vi "Configure Number of Points.vi"(8 "error in (no error)":errorcluster, 10 "Number of Point":i32, 11 "VNA-Ag87xx in":refnum<class "VNA-Ag87xx.lvclass">) -> (0 "error out":errorcluster, 3 "VNA-Ag87xx out":refnum<class "VNA-Ag87xx.lvclass">)   [LabVIEW 2020, in "VNA-Ag87xx.lvclass"]
doc: "Configures the number of points in the sweep.\nThe number of points will be choosen to the nearest supported."
uses:
  VNA-Ag87xx.lvclass
  C:/Sandbox/Git_Sandbox/WiSpry Test Framework source code (LV20)/WiSpry Test Framework/Instruments/Instrument.lvclass
  C:/Sandbox/Git_Sandbox/WiSpry Test Framework source code (LV20)/WiSpry Test Framework/Instruments/Vector Network Analyzer/Vector Network Analyzer.lvclass
  Instrument.lvclass/Instrument.ctl
  Vector Network Analyzer.lvclass/Vector Network Analyzer.ctl
  Instrument.lvclass
  Vector Network Analyzer.lvclass
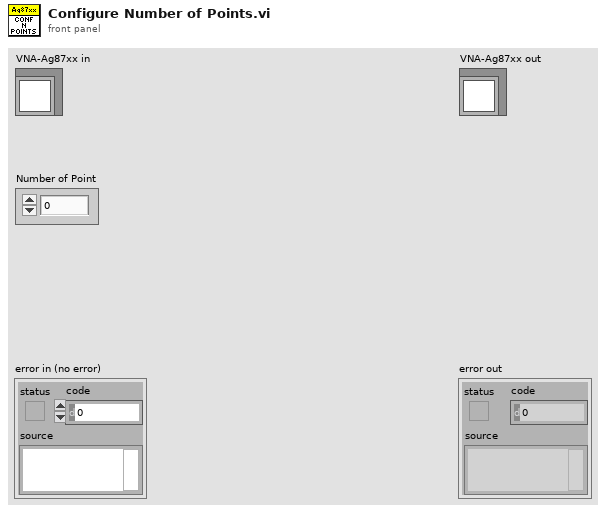
[diagram p1: front panel]
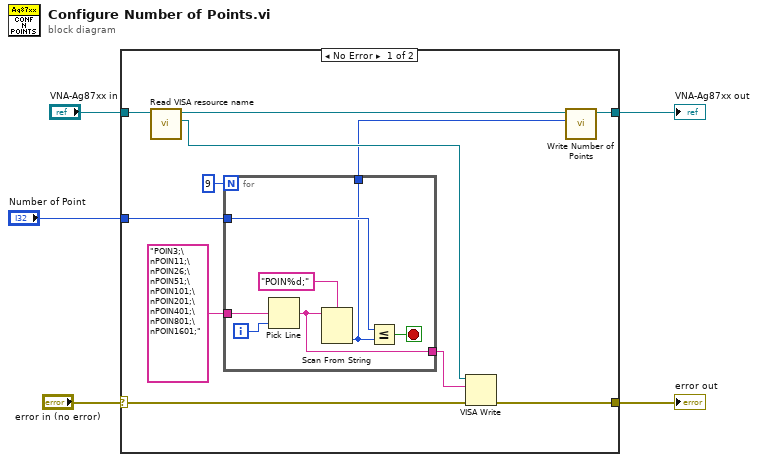
[diagram p0: block diagram]
diagram:
  n1 = case shown="No Error" "error in (no error)" {
    selector: "error in (no error)" -> [w13 w24]
    tunnel: [w10 w25] -> w3
    tunnel: "VNA-Ag87xx in" -> [w16 w25]
    tunnel: [w14 w24] -> w2
    tunnel: "Number of Point" -> [w9 _]
    frame No Error {
      n2 = call "Read VISA resource name.vi"("Instrument in"=w16) -> ("VISA resource name"=w12:refnum<visa-resource-name>, "Instrument out"=w11:refnum<class "VNA-Ag87xx.lvclass">)  [unwired: 9 in]
      n3 = for {
        N: 9 -> [_]
        tunnel: "POIN3;\nPOIN11;\nPOIN26;\nPOIN51;\nPOIN101;\nPOIN201;\nPOIN401;\nPOIN801;\nPOIN1601;" -> [w23]
        tunnel: w9 -> [w20]
        tunnel: [w17] -> w6
        tunnel: [w18] -> w7
        i -> [w22]
        stop <- w19 stop-if-true
        n4 = Pick Line(multi-line string=w23, line index=w22) -> (output string=w17:string)  [unwired: 1 in]
        n5 = Scan From String(format string="POIN%d;", input string=w17) -> (output 1=w18:i32)  [unwired: 3 in, 3 out]
        n6 = Less Or Equal?(x=w20, y=w18) -> (x <= y?=w19:bool)
      }
      n7 = VISA Write(VISA resource name=w12, write buffer=w6, error in (no error)=w13) -> (error out=w14:errorcluster)  [unwired: 2 out]
      n8 = call "Write Number of Points.vi"("Number of Points"=w7, "Vector Network Analyzer in"=w11) -> ("Vector Network Analyzer out"=w10:refnum<class "VNA-Ag87xx.lvclass">)  [unwired: 9 in]
    }
    frame Error {
    }
  }
  "error out" <- w2
  "VNA-Ag87xx out" <- w3
